vi "InfoStep.vi"(8 "error in":errorcluster, 10 "Seleziona Step":i32, 11 "Test Steps List":T1[](array[typedef])) -> (0 "error out":errorcluster, 3 "Info Test":string)   [LabVIEW 2019, in "ByteGSWebAPI.lvlib" / "ByteGSAPIBase.lvclass"]
doc: "Formatta le informazioni principali degli step in una info box più leggibile"
uses:
  ByteGSAPIBase.lvclass
  TypeDef/Step.ctl
  TypeDef/Asset.ctl
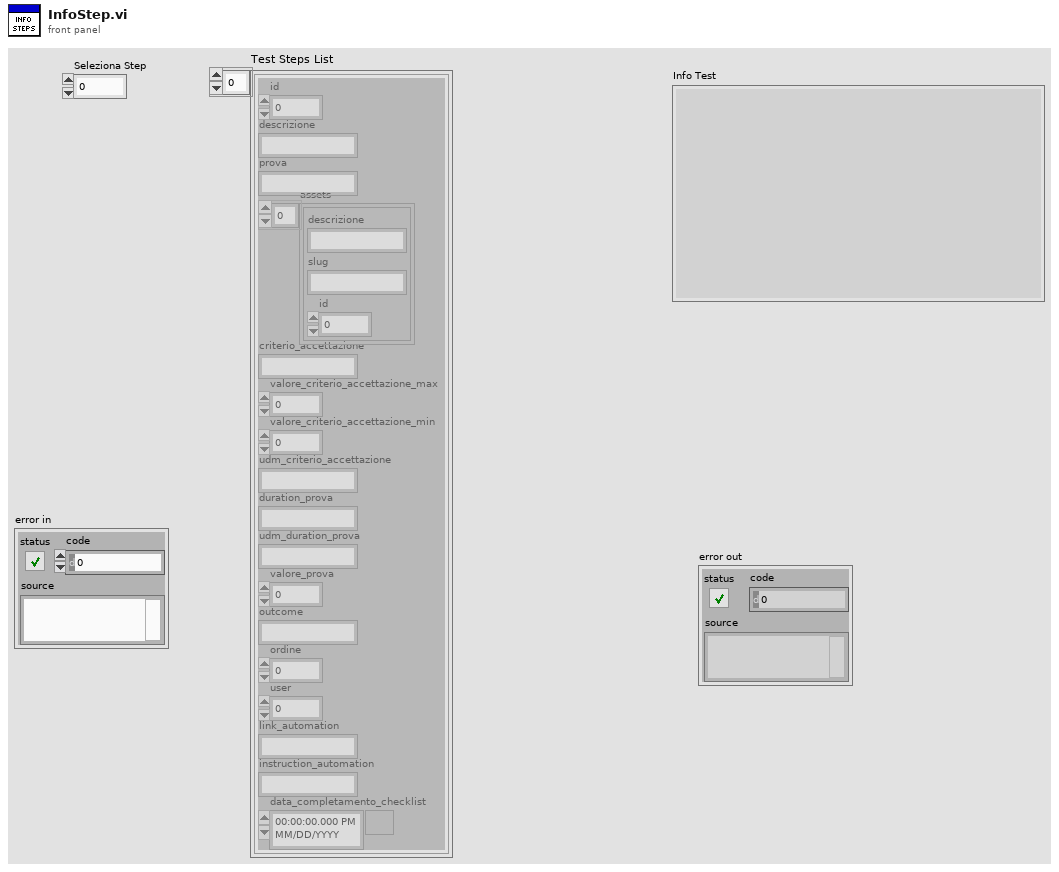
[diagram p1: front panel]
types:
  T1 = typedef "ByteGSWebAPI.lvlib/ByteGSAPIBase.lvclass/Step.ctl" = cluster{"id":i32, "descrizione":string, "prova":string, "assets":T2[], "criterio_accettazione":string, "valore_criterio_accettazione_max":dbl, "valore_criterio_accettazione_min":dbl, "udm_criterio_accettazione":string, "duration_prova":string, "udm_duration_prova":string, "valore_prova":dbl, "outcome":string, "ordine":i32, "user":i32, "link_automation":string, "instruction_automation":string, "data_completamento_checklist":timestamp}
  T2 = typedef "ByteGSWebAPI.lvlib/ByteGSAPIBase.lvclass/Asset.ctl" = cluster{"descrizione":string, "slug":string, "id":i32}
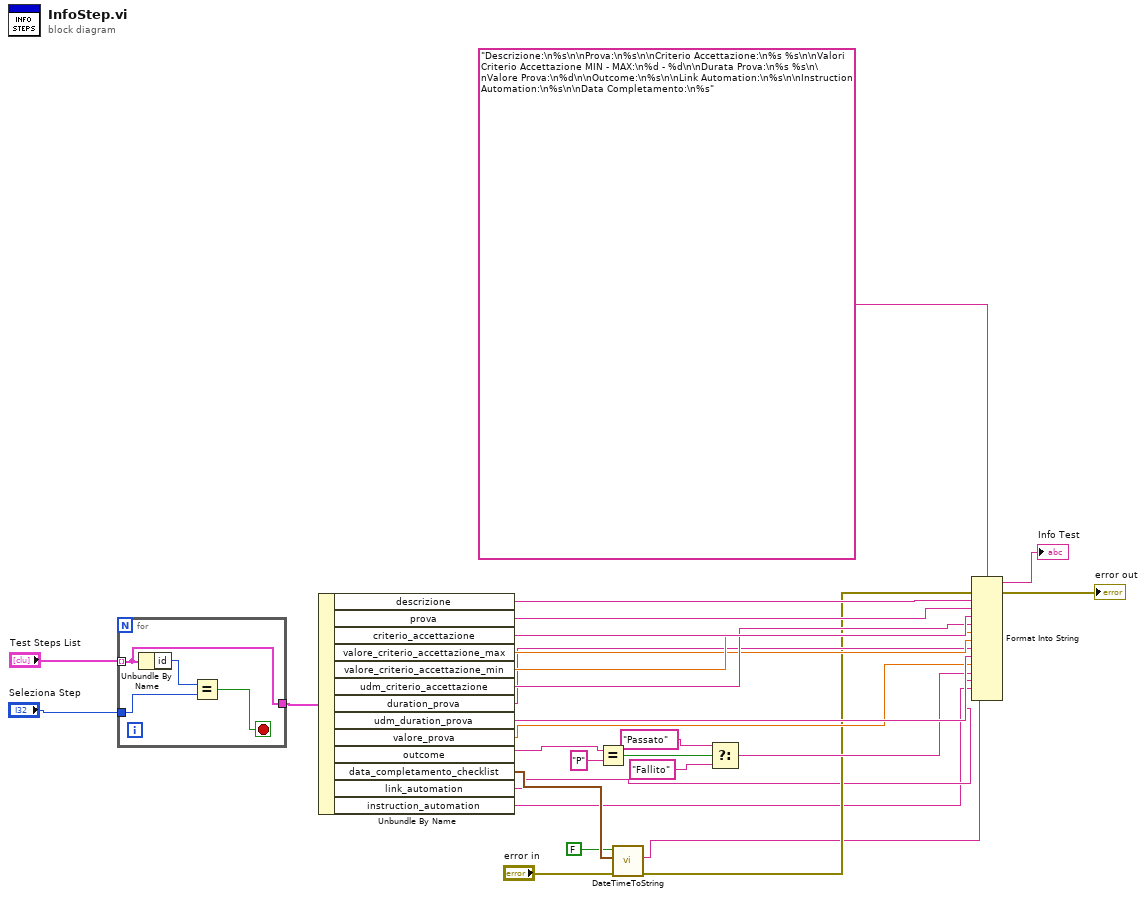
[diagram p0: block diagram]
diagram:
  n1 = for {
    tunnel: "Test Steps List" -> [w29] mode=indexing
    tunnel: "Seleziona Step" -> [w32]
    tunnel: [w29] -> w28
    stop <- w30 stop-if-true
    n2 = Unbundle By Name(w29) -> ("id"=w31:i32)
    n3 = Equal?(x=w31, y=w32) -> (x = y?=w30:bool)
  }
  n4 = Unbundle By Name(w28) -> ("descrizione"=w17:string, "prova"=w16:string, "criterio_accettazione"=w15:string, "valore_criterio_accettazione_max"=w12:dbl, "valore_criterio_accettazione_min"=w13:dbl, "udm_criterio_accettazione"=w14:string, "duration_prova"=w11:string, "udm_duration_prova"=w10:string, "valore_prova"=w9:dbl, "outcome"=w19:string, "data_completamento_checklist"=w25:timestamp, "link_automation"=w3:string, "instruction_automation"=w2:string)
  n5 = Equal?(x=w19, y="P") -> (x = y?=w21:bool)
  n6 = call "DateTimeToString.vi"("error in"="error in", "current time"=w25, "Time"=FALSE) -> ("error out"=w6:errorcluster, "Date string"=w1:string)  [unwired: 7 in]
  n7 = Select(t="Passato" ("y"), s=w21, f="Fallito" ("y")) -> (s? t:f=w8:string)
  n8 = Format Into String(format string="Descrizione:\n%s\n\nProva:\n%s\n\nCriterio Accettazione:\n%s %s\n\nValori Criterio Accettazione MIN - MAX:\n%d - %d\n\nDurata Prova:\n%s %s\n\nValore Prova:\n%d\n\nOutcome:\n%s\n\nLink Automation:\n%s\n\nInstruction Automation:\n%s\n\nData Completamento:\n%s", error in=w6, w17, w16, w15, w14, w13, w12, w11, w10, w9, w8, w3, w2, w1) -> (resulting string=→"Info Test":string, error out=→"error out":errorcluster)  [unwired: 1 in]
